vi "Normal.vi"(11 "Triangle":T2) -> (3 "Normal":T1)   [LabVIEW 2020, in "3D.lvlib"]
uses:
  3D.lvlib
  Triangle.ctl
  Vector 3D.ctl
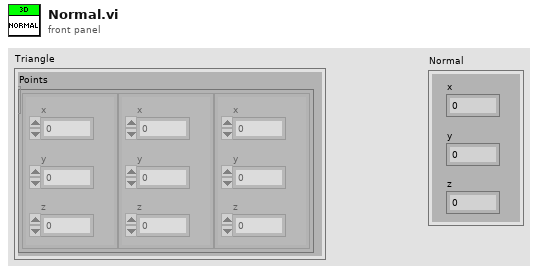
[diagram p1: front panel]
types:
  T1 = typedef "3D.lvlib/Vector 3D.ctl" = cluster{"x":sgl, "y":sgl, "z":sgl}
  T2 = typedef "3D.lvlib/Triangle.ctl" = cluster{"Points":T1[]}
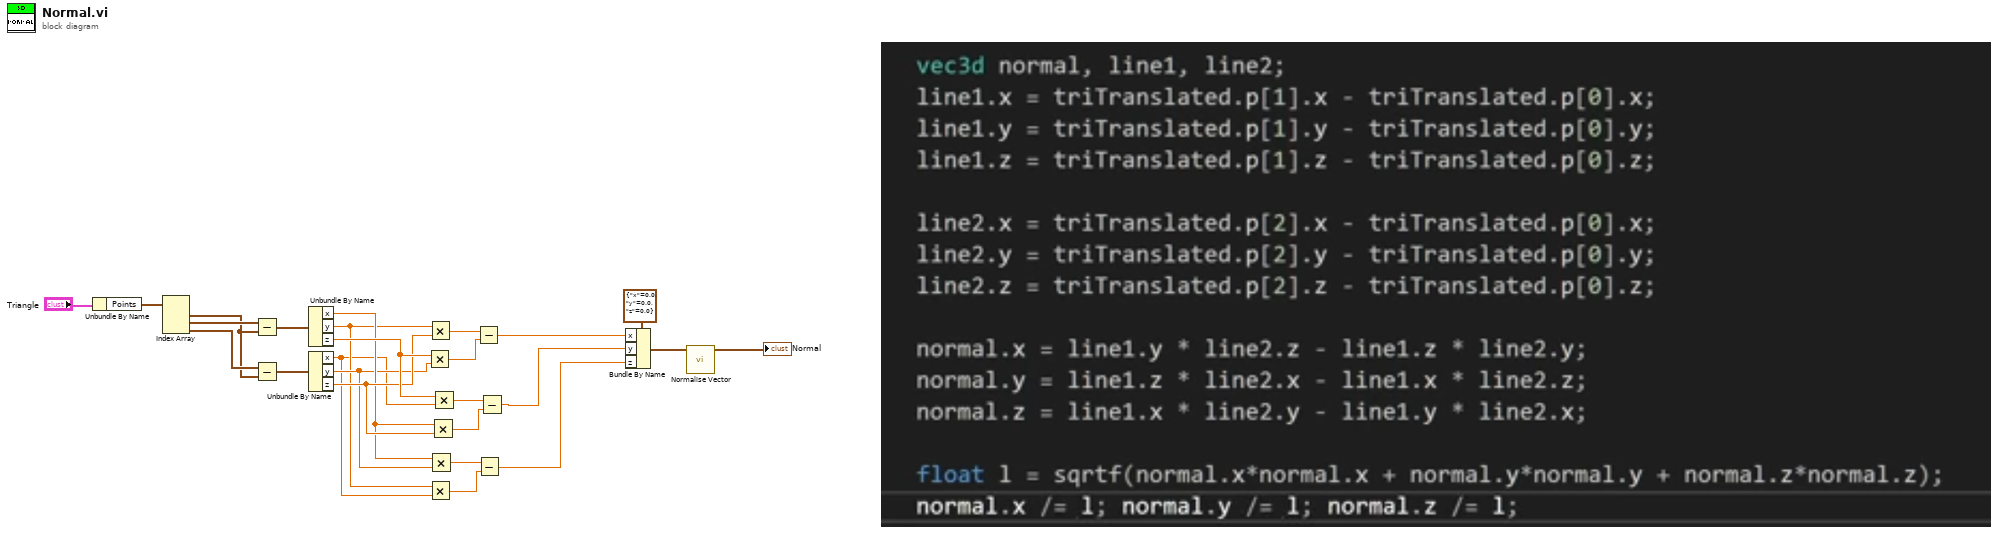
[diagram p0: block diagram]
diagram:
  n1 = Unbundle By Name("Triangle") -> ("Points"=w24:T1[])
  n2 = Index Array(array=w24) -> (element #1=w21:T1, element #2=w23:T1, element #3=w22:T1)  [unwired: 3 in]
  n3 = Subtract(x=w23, y=w21) -> (x-y=w19:T1)
  n4 = Subtract(x=w22, y=w21) -> (x-y=w18:T1)
  n5 = Unbundle By Name(w19) -> ("x"=w6:sgl, "y"=w4:sgl, "z"=w8:sgl)
  n6 = Unbundle By Name(w18) -> ("x"=w3:sgl, "y"=w5:sgl, "z"=w7:sgl)
  n7 = Multiply(x=w8, y=w5) -> (x*y=w16:sgl)
  n8 = Multiply(x=w4, y=w7) -> (x*y=w17:sgl)
  n9 = Multiply(x=w4, y=w3) -> (x*y=w11:sgl)
  n10 = Multiply(x=w6, y=w5) -> (x*y=w12:sgl)
  n11 = Multiply(x=w6, y=w7) -> (x*y=w14:sgl)
  n12 = Multiply(x=w8, y=w3) -> (x*y=w13:sgl)
  n13 = Subtract(x=w17, y=w16) -> (x-y=w15:sgl)
  n14 = Subtract(x=w12, y=w11) -> (x-y=w9:sgl)
  n15 = Subtract(x=w13, y=w14) -> (x-y=w10:sgl)
  n16 = Bundle By Name(cluster=T1 {"x"=0.0, "y"=0.0, "z"=0.0} ("Normal"), "x"=w15, "y"=w10, "z"=w9) -> (w2:T1)
  n17 = call "Normalise Vector.vi"("Vector 3D"=w2) -> ("Vector 3D Normalised"=→"Normal":T1)  [unwired: 10 in]
